vi "SD-Find Choice ID.vi"(8 "error in (no error)":errorcluster, 11 "Enum":string) -> (0 "error out":errorcluster, 3 "Choice ID":string)   [LabVIEW 2020]
doc: "This vi Search for choice id in database choice table and if not available then add Choice in table\nInput:\n1. Enum Items (eg. Test1,Test2,Test3 in this format)\n2. Error in\n\nOutput:\n1. Error out"
panel:
  out "subarray":string[](array[string])
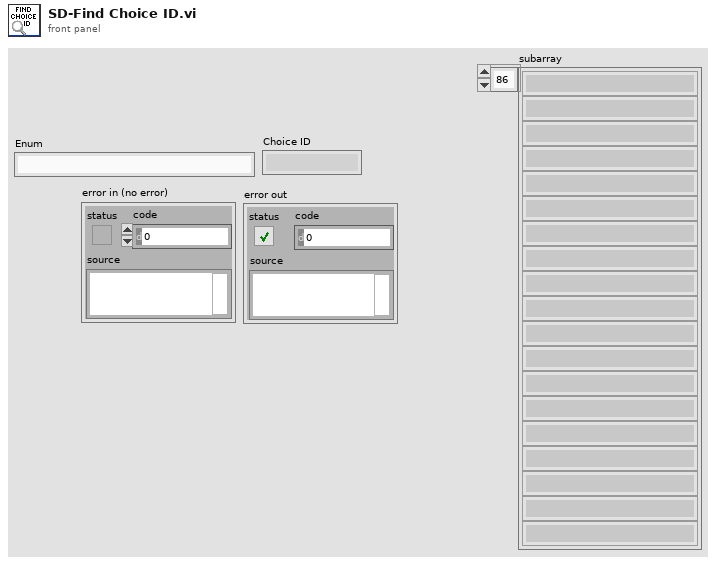
[diagram p1: front panel]
types:
  T1 = cluster{"Port":u16, "IP Address":string, "Authentication":cluster{"User":string, "Password":string, "Database":string}}
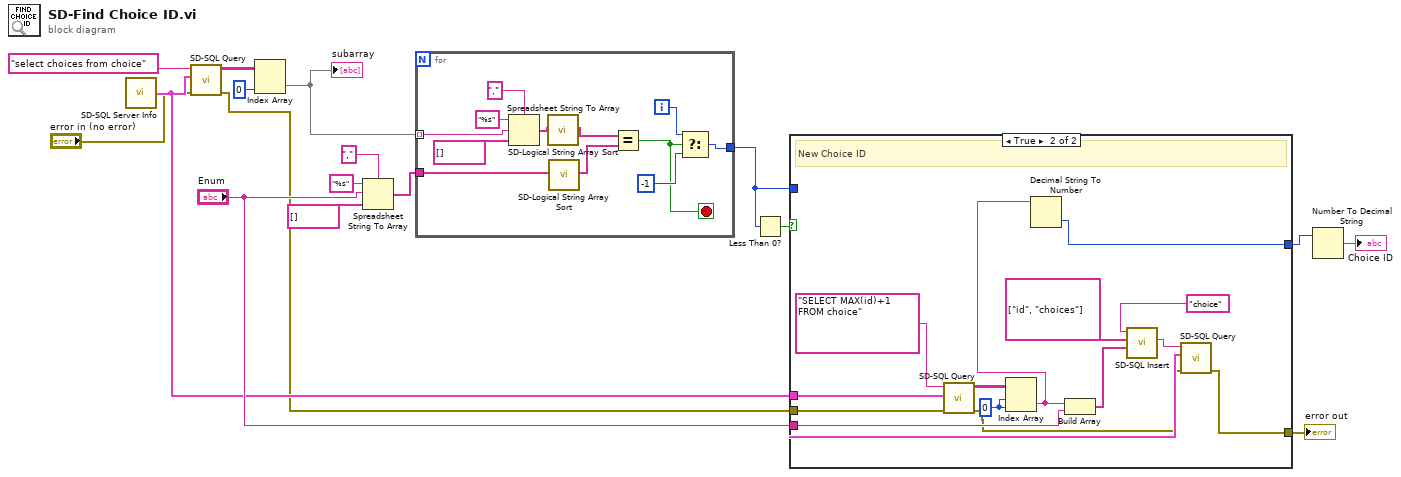
[diagram p0: block diagram]
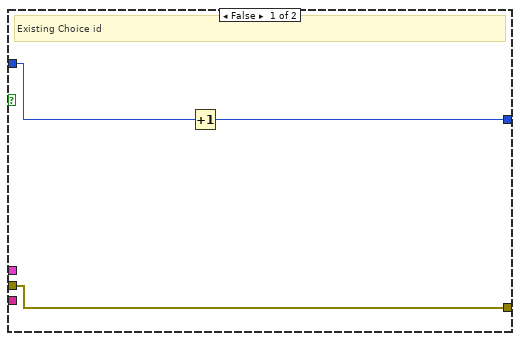
[diagram p2: hidden frame]
diagram:
  n1 = call "SD-SQL Server Info.vi"() -> ("SQL Server Info"=w10:T1)
  n2 = call "SD-SQL Query.vi"("error in (no error)"="error in (no error)", "SQL Server Info"=w10, "Query"="select choices from choice") -> ("error out"=w4:errorcluster, "data"=w15:string[][])  [unwired: 7 in]
  n3 = Index Array(array=w15, index (col)=0 ("disabled index (col)")) -> (element=w2:string[])  [unwired: 1 in]
  "subarray" <- w2
  n4 = Spreadsheet String To Array(delimiter (Tab)=",", format string="%s", spreadsheet string="Enum", array type (2D Dbl)=string[] []) -> (array=w1:string[])
  n5 = for {
    tunnel: w1 -> [w29]
    tunnel: w2 -> [w23] mode=indexing
    tunnel: [w19] -> w8
    i -> [w20]
    stop <- w18 stop-if-true
    n6 = Spreadsheet String To Array(delimiter (Tab)=",", format string="%s", spreadsheet string=w23, array type (2D Dbl)=string[] []) -> (array=w22:string[])
    n7 = call "SD-Logical String Array Sort.vi"("Unsorted List"=w22) -> ("Sorted List"=w27:string[])  [unwired: 18 in]
    n8 = call "SD-Logical String Array Sort.vi"("Unsorted List"=w29) -> ("Sorted List"=w28:string[])  [unwired: 18 in]
    n9 = Equal?(x=w27, y=w28) -> (x = y?=w18:bool)
    n10 = Select(t=w20, s=w18, f=-1 ("y")) -> (s? t:f=w19:i32)
  }
  n11 = Less Than 0?(x=w8) -> (x < 0?=w9:bool)
  n12 = case shown="True" w9 {
    tunnel: "Enum" -> [_ w40]
    tunnel: w10 -> [_ w38]
    tunnel: w8 -> [w32 _]
    tunnel: [w30 w33] -> w7
    tunnel: w4 -> [w31 w36]
    tunnel: [w31 w35] -> w3
    frame False {
      # "Existing Choice id"
      n13 = Increment(x=w32) -> (x+1=w30:i32)
    }
    frame True {
      w45 = 0 ("disabled index (col)")
      # "New Choice ID"
      n14 = call "SD-SQL Query.vi"("error in (no error)"=w36, "SQL Server Info"=w38, "Query"="SELECT MAX(id)+1 FROM choice") -> ("error out"=w34:errorcluster, "data"=w44:string[][])  [unwired: 7 in]
      n15 = Index Array(array=w44, index (row)=w45, index (col)=w45) -> (element=w37:string)
      n16 = Decimal String To Number(string=w37) -> (number=w33:i32)  [unwired: 2 in, 1 out]
      n17 = Build Array(w37, w40) -> (w39:string[])
      n18 = call "SD-SQL Insert.vi"("Values"=w39, "Column Names"=string[] ["id", "choices"], "Table"="choice") -> ("Query String"=w42:string)  [unwired: 8 in]
      n19 = call "SD-SQL Query.vi"("error in (no error)"=w34, "SQL Server Info"=w38, "Query"=w42) -> ("error out"=w35:errorcluster)  [unwired: 7 in, 1 out]
    }
  }
  "error out" <- w3
  n20 = Number To Decimal String(number=w7) -> (decimal integer string=→"Choice ID":string)  [unwired: 1 in]
